vi "8164B ReadOneLineResponse.vi"(8 "error in":errorcluster, 9 "timeout ms":i32=1000, 11 "KeySight 8164B control in":T1) -> (0 "error out":errorcluster, 2 "OneLineResponse":string, 3 "KeySight 8164B control out":T1)   [LabVIEW 2018, in "KeySight 8164B LAN InstrLib.lvlib"]
uses:
  KeySight 8164B LAN InstrLib.lvlib
  typedefs/KeySight 8164B control.ctl
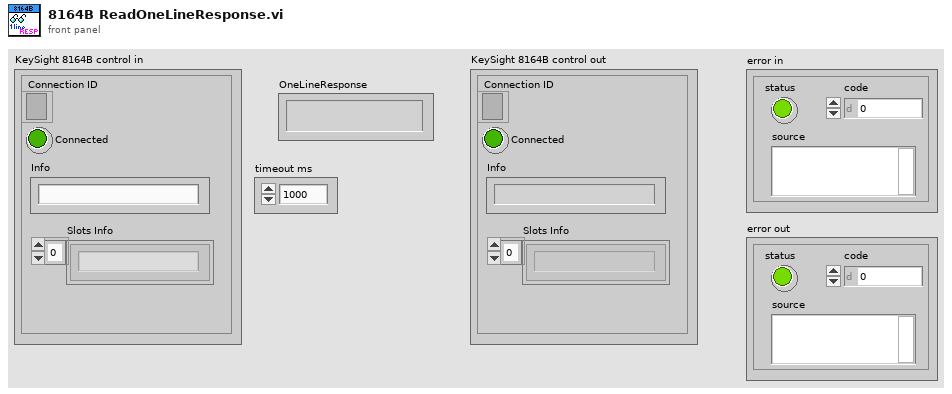
[diagram p1: front panel]
types:
  T1 = typedef "KeySight 8164B LAN InstrLib.lvlib/KeySight 8164B control.ctl" = cluster{"Connection ID":refnum<k5>, "Connected":bool, "Info":string, "Slots Info":string[]}
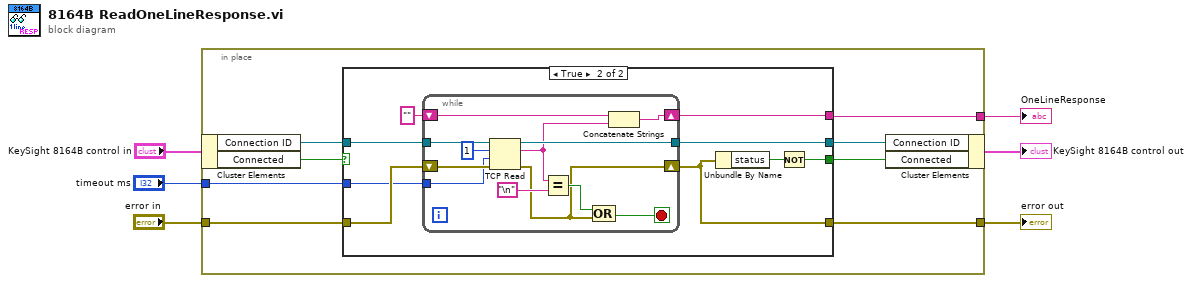
[diagram p0: block diagram]
diagram:
  n1 = in-place {
    in-place-border: "error in" -> [w12]
    in-place-border: [w11] -> w3
    in-place-border: [w10] -> w2
    in-place-border: "timeout ms" -> [w7]
    n2 = in-place-cluster #1("KeySight 8164B control in") -> ("Connection ID"=w13:refnum<k5>, "Connected"=w9:bool)
    n3 = case shown="True" w9 {
      selector: w9 -> [w16 _]
      tunnel: [w17 w26] -> w14
      tunnel: w13 -> [w17 w25]
      tunnel: w12 -> [w15 w24]
      tunnel: [w15 w23] -> w11
      tunnel: [_ w21] -> w10
      tunnel: [w16 w19] -> w8
      tunnel: w7 -> [_ w18]
      frame False {
      }
      frame True {
        n4 = while {
          tunnel: w25 -> [w38]
          tunnel: [w32] -> w26
          shift-right: [w31] -> w23
          shift-left: w24 -> [w36]
          shift-right: [w28] -> w21
          shift-left: "" -> [w30]
          tunnel: w18 -> [w27]
          stop <- w35 stop-if-true
          n5 = TCP Read(connection ID=w38, bytes to read=1, error in (no error)=w36, 9:w27) -> (connection ID out=w32:refnum<k5>, data out=w29:string, error out=w31:errorcluster)  [unwired: 1 in]
          n6 = Equal?(x=w29, y="\n") -> (x = y?=w33:bool)
          n7 = Compound Arithmetic op=OR(w33, w31) -> (w35:bool)
          n8 = Concatenate Strings(w30, w29) -> (w28:string)
        }
        n9 = Unbundle By Name(w23) -> ("status"=w20:bool)
        n10 = Not(x=w20) -> (.not. x?=w19:bool)
      }
    }
    n11 = in-place-cluster #1("Connection ID"=w14, "Connected"=w8) -> (→"KeySight 8164B control out":T1)
  }
  "error out" <- w3
  "OneLineResponse" <- w2
